vi "PathFinderWrap.vi"(8 "error in (no error)":errorcluster) -> (0 "error out":errorcluster)   [LabVIEW 2014]
uses:
  Controls/ShortestPath.ctl
  Libraries/Contact Data/Contact.ctl
  Libraries/Contact Data/Position.ctl
  Libraries/Contact Data/Controls.ctl
  Libraries/Contact Data/DestinationCluster.ctl
  Libraries/Contact Data/DesinationControls.ctl
  Libraries/Contact Data/PathData.ctl
  Libraries/Contact Data/Command.ctl
  Libraries/Map Data Folder/Map Data.lvlib
  Libraries/Contact Data/Contact Data.lvlib
panel:
  out "Array 2":T1[](array[typedef])
  out "Array":T7[][](array[typedef])
  out "Path":T7[](array[typedef])
  out "Current Pos":cluster{"Line Index":i32, "Line Pos Index":i32}
  out "Same Line +Dir?":bool
  out "Path Found?":bool
  out "Next Pos":cluster{"Line Index":i32, "Line Pos Index ":i32}
  out "Shortest Path":T7[](array[typedef])
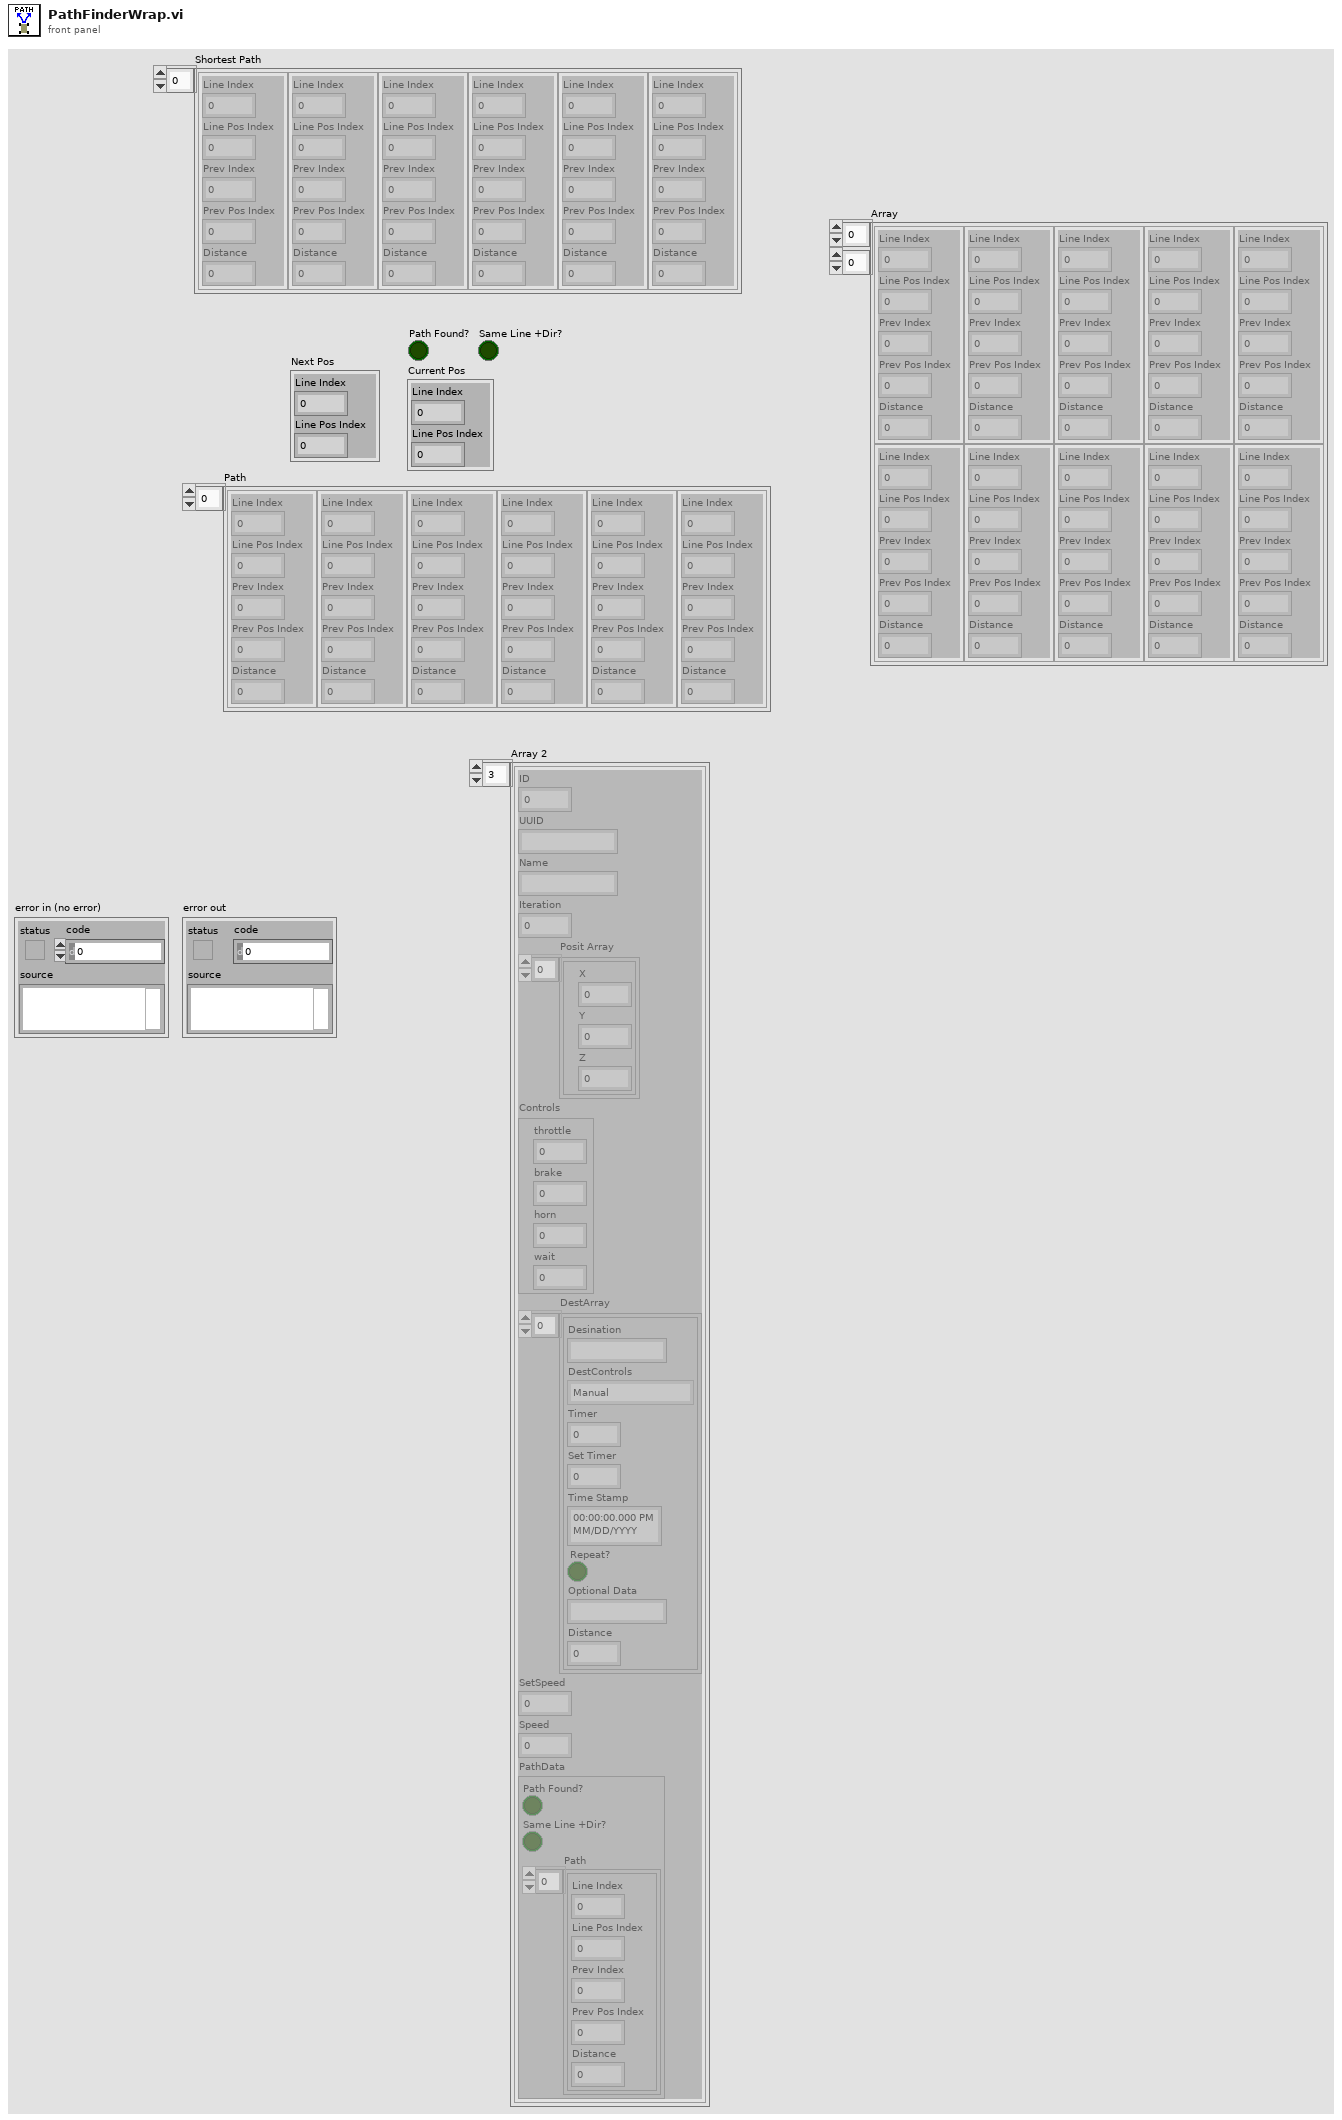
[diagram p1: front panel]
types:
  T1 = typedef "Contact Data.lvlib/Contact.ctl" = cluster{"ID":u32, "UUID":string, "Name":string, "Iteration":i32, "Posit Array":T2[], "Controls":T3, "DestArray":T4[], "SetSpeed":dbl, "Speed":dbl, "PathData":T6}
  T2 = typedef "Contact Data.lvlib/Position.ctl" = cluster{"X":dbl, "Y":dbl, "Z":dbl}
  T3 = typedef "Contact Data.lvlib/Controls.ctl" = cluster{"throttle":dbl, "brake":dbl, "horn":dbl, "wait":dbl}
  T4 = typedef "Contact Data.lvlib/DestinationCluster.ctl" = cluster{"Desination":string, "DestControls":T5, "Timer":u32, "Set Timer":u32, "Time Stamp":timestamp, "Repeat?":bool, "Optional Data":string, "Distance":dbl}
  T5 = typedef "Contact Data.lvlib/DesinationControls.ctl" = enum16{"Tracker", "Manual", "Stop", "Station DateTime", "Station Timer", "Maintain"}
  T6 = typedef "Contact Data.lvlib/PathData.ctl" = cluster{"Path Found?":bool, "Same Line +Dir?":bool, "Path":T7[]}
  T7 = typedef "ShortestPath.ctl" = cluster{"Line Index":i32, "Line Pos Index ":i32, "Prev Index ":i32, "Prev Pos Index":i32, "Distance":dbl}
  T8 = typedef "Map Data.lvlib/CursorList.ctl" = cluster{"Name":string, "Color":u32, "Style":u8, "Point Style":u8, "Name Visible":bool, "Allow Drag":bool, "Cursor Mode":u32, "Plot":i32, "Index":i32, "Position":cluster{"X":dbl, "Y":dbl}, "X Scale":u32, "Y Scale":u32, "Watch Plots":i32[], "Watch All Plots":bool, "Plot Area":i32, "Label Offset":cluster{"X":dbl, "Y":dbl}}[]
  T9 = typedef "Map Data.lvlib/All-Lines.ctl" = T10[]
  T10 = typedef "Map Data.lvlib/LineCluster.ctl" = cluster{"Line name":string, "Line array":cluster{"X":dbl, "Y":dbl, "Z":dbl}[], "Line connections":T11[]}
  T11 = typedef "Map Data.lvlib/LineConnection.ctl" = cluster{"Index":i32, "Switch Pos":cluster{"X":dbl, "Y":dbl, "Z":dbl}, "Switch operational":bool, "Switch State":bool, "Connection Index":i32, "Connection Pos":cluster{"X":dbl, "Y":dbl, "Z":dbl}, "LinePos Index":i32, "ConnectPos Index":i32, "Same direction?":bool, "Manual Overide":bool, "Manual State":bool}
  T12 = typedef "Contact Data.lvlib/Command.ctl" = enum16{"Set All Contacts", "Load", "Save", "Get All Data", "Get Single Data (ID)", "Get Single Data", "Set Position", "Set Single Path", "Set Destinations", "Set Controls", "Remove Single Data", "Remove UUID Contact", "Set Single ALL", "Is Data Modified", "Import Data"}
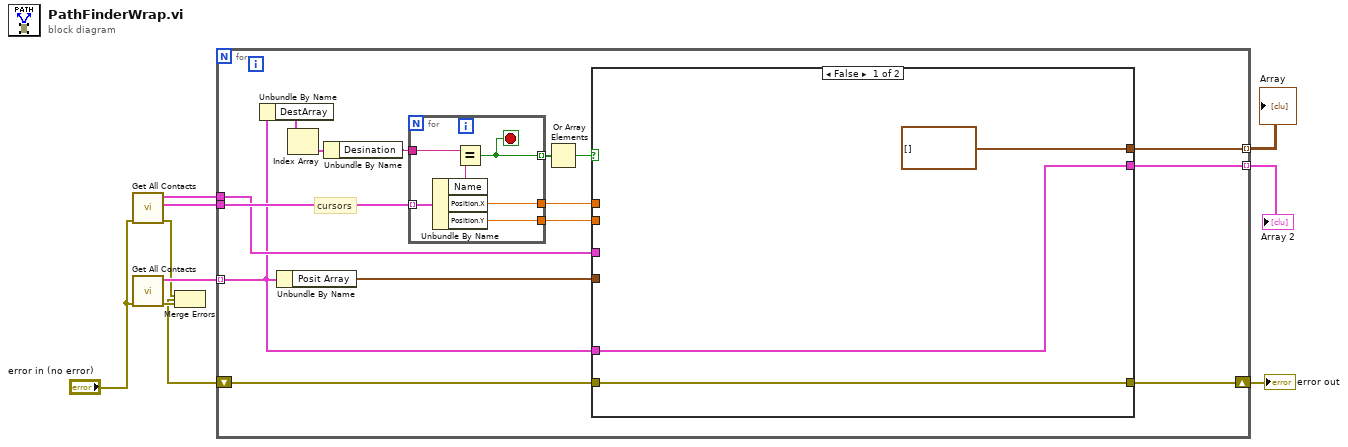
[diagram p0: block diagram]
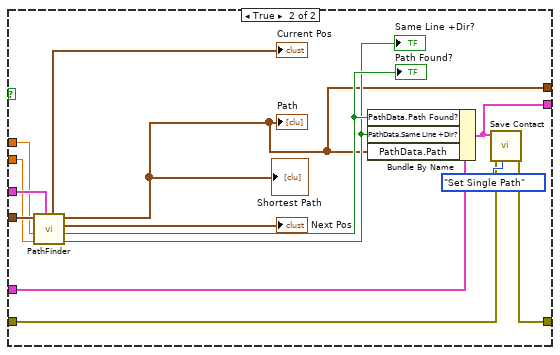
[diagram p2: hidden frame]
diagram:
  n1 = call "Get All Contacts.vi"("error in (no error)"="error in (no error)") -> ("error out"=w3:errorcluster, "Cursor List"=w8:T8, "All Lines out"=w9:T9)  [unwired: 8 in]
  n2 = call "Get All Contacts.vi"("error in (no error)"="error in (no error)") -> ("error out"=w4:errorcluster, "Contacts"=w10:T1[])  [unwired: 9 in]
  n3 = Merge Errors(w3, w4) -> (w2:errorcluster)
  n4 = for {
    tunnel: w10 -> [w15] mode=indexing
    tunnel: w9 -> [w19]
    tunnel: w8 -> [w21]
    tunnel: [w14] -> w5 mode=indexing
    tunnel: [w13] -> w6 mode=indexing
    shift-right: [w11] -> w1
    shift-left: w2 -> [w12]
    # "cursors"
    n5 = Unbundle By Name(w15) -> ("DestArray"=w25:T4[])
    n6 = Unbundle By Name(w15) -> ("Posit Array"=w20:T2[])
    n7 = Index Array(array=w25) -> (element=w24:T4)  [unwired: 1 in]
    n8 = Unbundle By Name(w24) -> ("Desination"=w23:string)
    n9 = for {
      tunnel: w23 -> [w44]
      tunnel: w21 -> [w43] mode=indexing
      tunnel: [w47] -> w17
      tunnel: [w46] -> w18
      tunnel: [w45] -> w22 mode=indexing
      stop <- w45 stop-if-true
      n10 = Unbundle By Name(w43) -> ("Name"=w48:string, "Position.X"=w46:dbl, "Position.Y"=w47:dbl)
      n11 = Equal?(x=w44, y=w48) -> (x = y?=w45:bool)
    }
    n12 = Or Array Elements(Boolean array=w22) -> (logical OR=w16:bool)
    n13 = case shown="False" w16 {
      tunnel: w20 -> [_ w42]
      tunnel: w19 -> [_ w41]
      tunnel: w18 -> [_ w40]
      tunnel: w17 -> [_ w39]
      tunnel: w15 -> [w28 w35]
      tunnel: [w28 w32] -> w14
      tunnel: [T7[] [] ("Shortest Path") w29] -> w13
      tunnel: [w27 w31] -> w11
      tunnel: w12 -> [w27 w30]
      frame False {
      }
      frame True {
        n14 = call "PathFinder.vi"("All Lines"=w41, "Target Z"=w39, "Target X"=w40, "Posit Array"=w42) -> ("Same Line +Dir?"=w33:bool, "Path Found?"=w34:bool, "Next Pos"=→"Next Pos":cluster{"Line Index":i32, "Line Pos Index ":i32}, "Shortest Path"=w29:T7[], "Current Pos"=→"Current Pos":cluster{"Line Index":i32, "Line Pos Index":i32})  [unwired: 2 in, 1 out]
        "Same Line +Dir?" <- w33
        "Shortest Path" <- w29
        "Path Found?" <- w34
        "Path" <- w29
        n15 = Bundle By Name(cluster=w35, "PathData.Path Found?"=w34, "PathData.Same Line +Dir?"=w33, "PathData.Path"=w29) -> (w32:T1)
        n16 = call "Save Contact.vi"("Command"=Command."Set Single Path", "error in (no error)"=w30, "Contact"=w32) -> ("error out"=w31:errorcluster)  [unwired: 7 in, 1 out]
      }
    }
  }
  "Array" <- w6
  "Array 2" <- w5
  "error out" <- w1
